vi "Practica 7.vi"() -> ()   [LabVIEW 2018]
uses:
  <vilib>/LabVIEW Interface for Arduino/Type Defs/Digital Pin.ctl
  <vilib>/LabVIEW Interface for Arduino/Type Defs/Pin Mode.ctl
  <vilib>/LabVIEW Interface for Arduino/LabVIEW Interface for Arduino.lvlib
  <vilib>/ptbypt/NI_PtbyPt.lvlib
panel:
  in  "Puesta a 0":bool
  in  "stop":bool
  out "Contador":dbl
  out "Impulso":bool
  in  "Seleccion de PIN":T1
  # "Practica 7:Contador de Impulsos \nen una Entrada Digital"
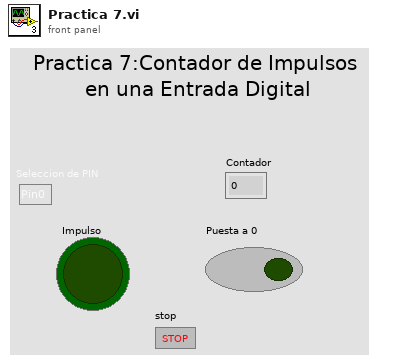
[diagram p1: front panel]
types:
  T1 = typedef "LabVIEW Interface for Arduino.lvlib/Digital Pin.ctl" = enum8{"Pin0", "Pin1", "Pin2", "Pin3", "Pin4", "Pin5", "Pin6", "Pin7", "Pin8", "Pin9", "Pin10", "Pin11", "Pin12", "Pin13"}
  T2 = typedef "LabVIEW Interface for Arduino.lvlib/Arduino Resource.ctl" = cluster{"VISA resource":refnum<visa-resource-name>, "Board Type":T3, "Connection Type":enum8{"USB / Serial"}, "Bytes Per Packet (15)":u8}
  T3 = typedef "LabVIEW Interface for Arduino.lvlib/Board Type.ctl" = enum16{"Uno", "Dimuelanove w/Atmega 328", "Mega 2560"}
  T4 = typedef "LabVIEW Interface for Arduino.lvlib/Pin Mode.ctl" = enum8{"Input", "Output"}
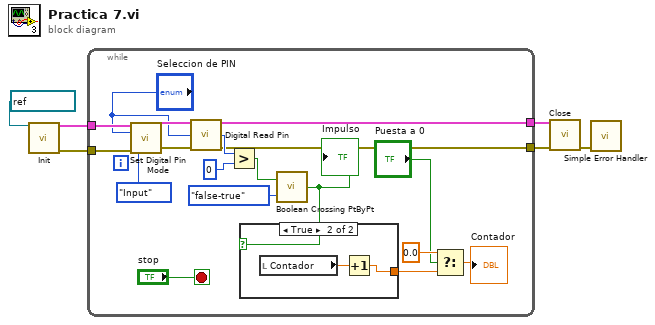
[diagram p0: block diagram]
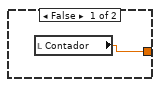
[diagram p2: hidden frame]
diagram:
  n1 = call <vilib>:"Init.vi"("VISA resource"=refnum<visa-resource-name> "COM9") -> ("Arduino Resource"=w5:T2, "error out"=w4:errorcluster)  [unwired: 17 in]
  n2 = while {
    tunnel: w5 -> [w23]
    tunnel: w4 -> [w22]
    tunnel: [w13] -> w2
    tunnel: [w12] -> w1
    stop <- "stop" stop-if-true
    n3 = call <vilib>:"Set Digital Pin Mode.vi"("Arduino Resource"=w23, "Digital I/O Pin"="Seleccion de PIN", "Pin Mode (Input)"=Pin_Mode."Input", "error in"=w22) -> ("Arduino Resource"=w20:T2, "error out"=w21:errorcluster)  [unwired: 10 in]
    n4 = call <vilib>:"Digital Read Pin.vi"("Arduino Resource"=w20, "Digital I/O Pin (0)"="Seleccion de PIN", "error in"=w21) -> ("Arduino Resource"=w12:T2, "Value"=w17:u8, "error out"=w13:errorcluster)  [unwired: 10 in]
    n5 = Greater?(x=w17, y=0) -> (0:w15:bool)
    n6 = call <vilib>:"Boolean Crossing PtByPt.vi"("direction"=enum16{"either", "false-true", "true-false"}."false-true", "input"=w15) -> ("crossing"=w11:bool)  [unwired: 1 in]
    "Impulso" <- w11
    n7 = case shown="True" w11 {
      tunnel: [w25 w27] -> w10
      frame False {
        n8 = local read "Contador"() -> (w25:dbl)
      }
      frame True {
        n9 = local read "Contador"() -> (w26:dbl)
        n10 = Increment(x=w26) -> (x+1=w27:dbl)
      }
    }
    n11 = Select(t=0.0, s="Puesta a 0", f=w10) -> (s? t:f=→"Contador":dbl)
  }
  n12 = call <vilib>:"Close.vi"("Arduino Resource"=w1, "error in"=w2) -> ("error out"=w3:errorcluster)  [unwired: 13 in]
  n13 = call <vilib>:"Simple Error Handler.vi"("error in (no error)"=w3) -> ()  [unwired: 4 in, 5 out]
